vi "Sensor Data.vi"() -> ()   [LabVIEW 2015]
panel:
  out "IMU Heading":dbl
  out "Gyro Heading":dbl
  out "Right Grabber Position":dbl
  out "Left Grabber Position":dbl
  out "Right Catapult Limit Switch":bool
  out "Climb Arm Deploy Motor":dbl
  out "Catapult Winch Motor":dbl
  out "Ball Lifter Left":dbl
  out "Ball Lifter Right":dbl
  out "Left Master":dbl
  out "Right Master":dbl
  out "Left Catapult Limit Switch":bool
  out "Forward IR Sensor":dbl
  out "Left IR Sensor":bool
  out "Right IR Sensor":bool
  out "Robot Heading":dbl
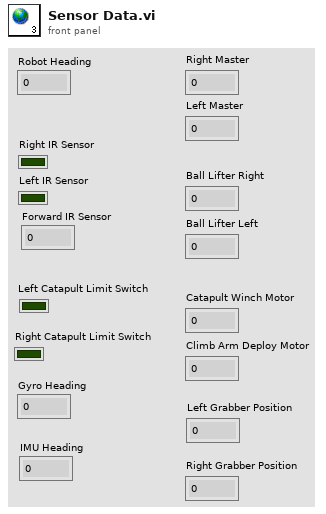
[diagram p1: front panel]
diagram:
